vi "ConvertToFXP.vi"(11 "Digtal":bool[][](array[boolean])) -> (3 "FXP":fxp<+,20,20>[](array[numeric]))   [LabVIEW 2019]
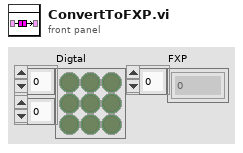
[diagram p1: front panel]
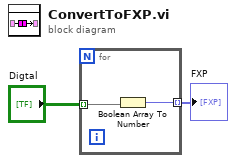
[diagram p0: block diagram]
diagram:
  n1 = for {
    tunnel: "Digtal" -> [w4] mode=indexing
    tunnel: [w3] -> w1 mode=indexing
    n2 = Boolean Array To Number ("布尔数组至数值转换")(Boolean array=w4) -> (number=w3:fxp<+,20,20>)
  }
  "FXP" <- w1
